vi "OutputNoteHandling.vi"   [LabVIEW 2023]
doc: "This VI sends commands to the arm subsystem."
uses:
  <vilib>/Rock Robotics/WPI/ThirdParty/REV Robotics/REVLib/Typedef/Spark MAX Limit Direction.ctl
  GlobalNoteHandling.vi
  GRNF_Kraken.vi
  GRNF_GenericMotor.vi
  GRNF_Servo.vi
types:
  T1 = typedef "Spark MAX Limit Direction.ctl" = enum16{"Forward Limit", "Reverse Limit"}
  T2 = typedef "Spark MAX Limit Switch Polarity.ctl" = enum16{"Normally Open", "Normally Closed"}
  T3 = typedef "WPI_ServoDeviceRef.ctl" = cluster{"DeviceStatus":errorcluster, "PWM Channel":T4, "DeadBand":T5}
  T4 = typedef "FPGA_DIOPWMChannel.ctl" = enum8{"PWM 0", "PWM 1", "PWM 2", "PWM 3", "PWM 4", "PWM 5", "PWM 6", "PWM 7", "PWM 8", "PWM 9", "PWM MXP 0", "PWM MXP 1", "PWM MXP 2", "PWM MXP 3", "PWM MXP 4", "PWM MXP 5", "PWM MXP 6", "PWM MXP 7", "PWM MXP 8", "PWM MXP 9", "Invalid"}
  T5 = typedef "WPI_PWMDeadband.ctl" = cluster{"Name":string, "maxPositivePwm":i32, "minPositivePwm":i32, "centerPwm":i32, "maxNegativePwm":i32, "minNegativePwm":i32, "angularRange":u16}
  T6 = enum16{"No Changed Output", "New Normal Output", "New Testing Output"}
  T7 = typedef "WPI_MotorControlDeviceRef.ctl" = cluster{"DeviceStatus":errorcluster, "Type":T8, "PWM":cluster{"PWM Channel":T4, "DeadBand":T5}, "CAN":cluster{"Device Number":u8, "SetOutput VI Ref":variant, "GetOutput VI Ref":variant, "Enable VI Ref":variant, "Disable VI Ref":variant, "Data":variant}, "Invert":bool, "DIO PWM":cluster{"PWM \"Enable\" Channel":T4, "DIOChannel":T9, "PWM Rate":dbl}}
  T8 = typedef "WPI_MotorControlType.ctl" = enum16{"PWM", "CAN", "DIO PWM"}
  T9 = typedef "FPGA_DIOChannel.ctl" = enum8{"DIO 0", "DIO 1", "DIO 2", "DIO 3", "DIO 4", "DIO 5", "DIO 6", "DIO 7", "DIO 8", "DIO 9", "DIO MXP 0", "DIO MXP 1", "DIO MXP 2", "DIO MXP 3", "DIO MXP 4", "DIO MXP 5", "DIO MXP 6", "DIO MXP 7", "DIO MXP 8", "DIO MXP 9", "DIO MXP 10", "DIO MXP 11", "DIO MXP 12", "DIO MXP 13", "DIO MXP 14", "DIO MXP 15", "SPI Port CS1", "SPI Port CS2", "SPI Port CS3", "SPI Port MISO", "SPI Port MOSI", "Invalid"}
  T10 = typedef "DeviceReference.ctl" = cluster{"CANbus Name":string, "Device Encoding":u32, "Device Name":string}
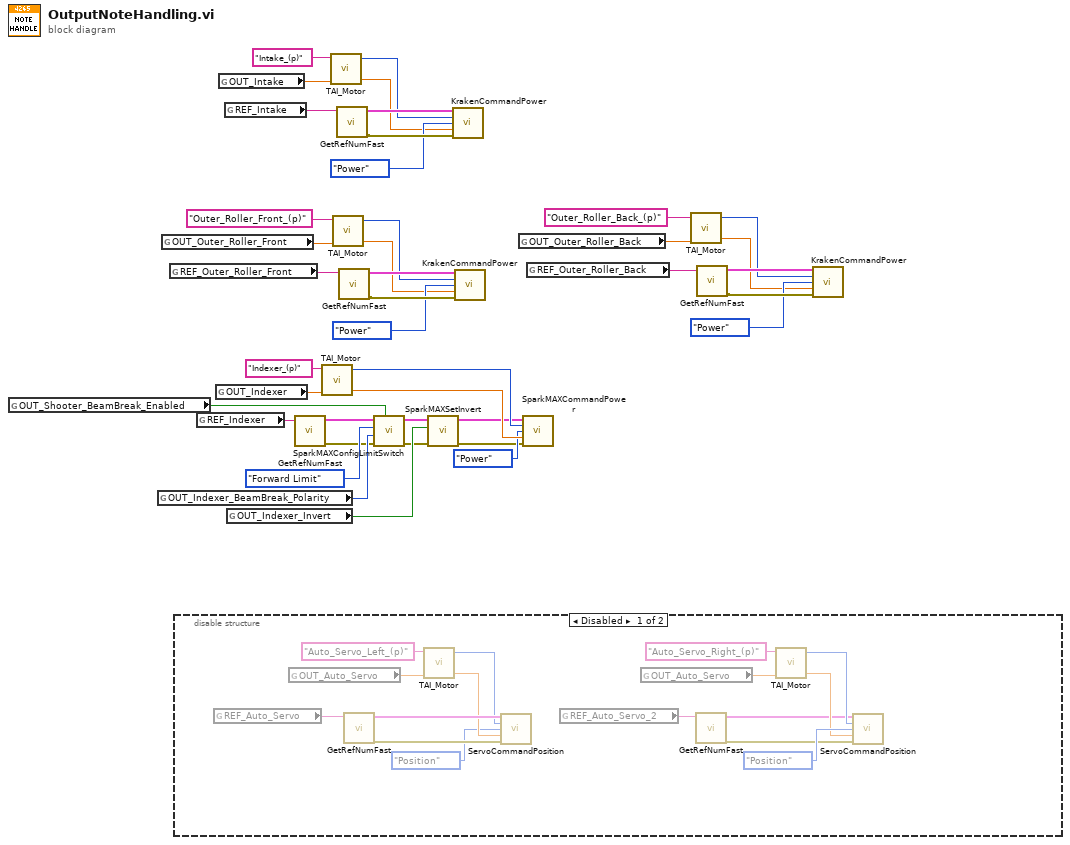
[diagram p0: block diagram]
diagram:
  n1 = global read "GlobalNoteHandling.vi" "OUT_Shooter_BeamBreak_Enabled"() -> (w32:bool)
  n2 = global read "GlobalNoteHandling.vi" "OUT_Indexer_BeamBreak_Polarity"() -> (w34:T2)
  n3 = global read "GlobalNoteHandling.vi" "OUT_Outer_Roller_Front"() -> (w20:dbl)
  n4 = global read "GlobalNoteHandling.vi" "REF_Outer_Roller_Front"() -> (w21:string)
  n5 = disable-structure shown="Disabled" {
    frame Disabled {
      n6 = global read "GlobalNoteHandling.vi" "REF_Auto_Servo"() -> (w55:string)
      n7 = global read "GlobalNoteHandling.vi" "OUT_Auto_Servo"() -> (w54:dbl)
      n8 = call-poly "GetRefNumFast.vi"("RefNum Name"=w55) -> ("Error"=w52:errorcluster, "Device Reference"=w53:T3)  [unwired: 5 in]
      n9 = call "TAI_Motor.vi"("Normal Output"=w54, "Actuator Name"="Auto_Servo_Left_(p)") -> ("Interlocked Output"=w50:dbl, "Testing Mode"=w51:T6)  [unwired: 3 in]
      n10 = call "ServoCommandPosition.vi"("Device Reference"=w53, "Output Mode"=w51, "Control Mode"=enum16{"Safety", "Position"}."Position", "Power or Testing Power"=w50, "Error (in)"=w52) -> ()  [unwired: 11 in]
      n11 = global read "GlobalNoteHandling.vi" "REF_Auto_Servo_2"() -> (w42:string)
      n12 = global read "GlobalNoteHandling.vi" "OUT_Auto_Servo"() -> (w43:dbl)
      n13 = call-poly "GetRefNumFast.vi"("RefNum Name"=w42) -> ("Error"=w45:errorcluster, "Device Reference"=w44:T3)  [unwired: 5 in]
      n14 = call "TAI_Motor.vi"("Normal Output"=w43, "Actuator Name"="Auto_Servo_Right_(p)") -> ("Interlocked Output"=w47:dbl, "Testing Mode"=w46:T6)  [unwired: 3 in]
      n15 = call "ServoCommandPosition.vi"("Device Reference"=w44, "Output Mode"=w46, "Control Mode"=enum16{"Safety", "Position"}."Position", "Power or Testing Power"=w47, "Error (in)"=w45) -> ()  [unwired: 11 in]
    }
    frame Enabled {
    }
  }
  n16 = global read "GlobalNoteHandling.vi" "REF_Indexer"() -> (w35:string)
  n17 = global read "GlobalNoteHandling.vi" "OUT_Indexer"() -> (w39:dbl)
  n18 = global read "GlobalNoteHandling.vi" "OUT_Intake"() -> (w5:dbl)
  n19 = global read "GlobalNoteHandling.vi" "REF_Intake"() -> (w4:string)
  n20 = global read "GlobalNoteHandling.vi" "OUT_Indexer_Invert"() -> (w31:bool)
  n21 = call-poly "GetRefNumFast.vi"("RefNum Name"=w35) -> ("Error"=w29:errorcluster, "Device Reference"=w30:T7)  [unwired: 5 in]
  n22 = call "TAI_Motor.vi"("Normal Output"=w39, "Actuator Name"="Indexer_(p)") -> ("Interlocked Output"=w38:dbl, "Testing Mode"=w37:T6)  [unwired: 3 in]
  n23 = call "TAI_Motor.vi"("Normal Output"=w5, "Actuator Name"="Intake_(p)") -> ("Interlocked Output"=w1:dbl, "Testing Mode"=w8:T6)  [unwired: 3 in]
  n24 = call "TAI_Motor.vi"("Normal Output"=w20, "Actuator Name"="Outer_Roller_Front_(p)") -> ("Interlocked Output"=w22:dbl, "Testing Mode"=w24:T6)  [unwired: 3 in]
  n25 = call-poly "GetRefNumFast.vi"("RefNum Name"=w4) -> ("Error"=w9:errorcluster, "Device Reference"=w10:T10)  [unwired: 5 in]
  n26 = call-poly "GetRefNumFast.vi"("RefNum Name"=w21) -> ("Error"=w25:errorcluster, "Device Reference"=w26:T10)  [unwired: 5 in]
  n27 = call "SparkMAXConfigLimitSwitch.vi"("Enabled?"=w32, "Error (in)"=w29, "Polarity"=w34, "fwd/rev limit"=Spark_MAX_Limit_Direction."Forward Limit" ("Limit Switch"), "Device Reference (in)"=w30) -> ("Error (out)"=w2:errorcluster, "Device Reference (out)"=w3:T7)  [unwired: 3 in]
  n28 = call "SparkMAXSetInvert.vi"("Error (in)"=w2, "Inverted?"=w31, "Device Reference (in)"=w3) -> ("Error (out)"=w28:errorcluster, "Device Reference (out)"=w27:T7)  [unwired: 5 in]
  n29 = call "KrakenCommandPower.vi"("Device Reference (in)"=w10, "Output Mode"=w8, "Control Mode"=enum16{"Safety", "Power"}."Power", "Power or Testing Power"=w1, "Error (in)"=w9) -> ()  [unwired: 11 in]
  n30 = call "KrakenCommandPower.vi"("Device Reference (in)"=w26, "Output Mode"=w24, "Control Mode"=enum16{"Safety", "Power"}."Power", "Power or Testing Power"=w22, "Error (in)"=w25) -> ()  [unwired: 11 in]
  n31 = global read "GlobalNoteHandling.vi" "OUT_Outer_Roller_Back"() -> (w12:dbl)
  n32 = call "SparkMAXCommandPower.vi"("Device Reference (in)"=w27, "Output Mode"=w37, "Control Mode"=enum16{"Safety", "Power"}."Power", "Power or Testing Power"=w38, "Error (in)"=w28) -> ()  [unwired: 11 in]
  n33 = global read "GlobalNoteHandling.vi" "REF_Outer_Roller_Back"() -> (w11:string)
  n34 = call "TAI_Motor.vi"("Normal Output"=w12, "Actuator Name"="Outer_Roller_Back_(p)") -> ("Interlocked Output"=w14:dbl, "Testing Mode"=w16:T6)  [unwired: 3 in]
  n35 = call-poly "GetRefNumFast.vi"("RefNum Name"=w11) -> ("Error"=w17:errorcluster, "Device Reference"=w18:T10)  [unwired: 5 in]
  n36 = call "KrakenCommandPower.vi"("Device Reference (in)"=w18, "Output Mode"=w16, "Control Mode"=enum16{"Safety", "Power"}."Power", "Power or Testing Power"=w14, "Error (in)"=w17) -> ()  [unwired: 11 in]
